vi "diagnose_status.vi"(5 "RMS mismatch":sgl, 7 "Repair count":i32, 8 "Axis positions":sgl[][](array[numeric]), 9 "Sum amplitudes":sgl[][](array[numeric]), 11 "Match error":sgl[](array[numeric])) -> (0 "Position valid":bool)   [LabVIEW 2014]
panel:
  in  "Warn RMS mismatch (volts)":sgl=0.015 format="%#_3p"
  in  "Max RMS mismatch (volts)":sgl=0.03 format="%#_3p"
  in  "Max repair count":i32=30
  in  "Max axis position":sgl=0.75
  in  "Max match error":sgl=500.0
  in  "Min amplitude":sgl=0.02
  # "Parameters:"
  # "This sets the maximum acceptable matching error between the two rays (in microns)."
  # "If impulse repair count or RMS mismatch (signal + noise) exceeds these thresholds on a single block, then the status is invalid."
  # "This sets the minimum acceptable signal amplitude."
  # "This sets the maximum acceptable axis position as a fraction of full scale."
  # "We warn if there are any impulse repairs or if the max per-block RMS mismatch exceeds this threshold."
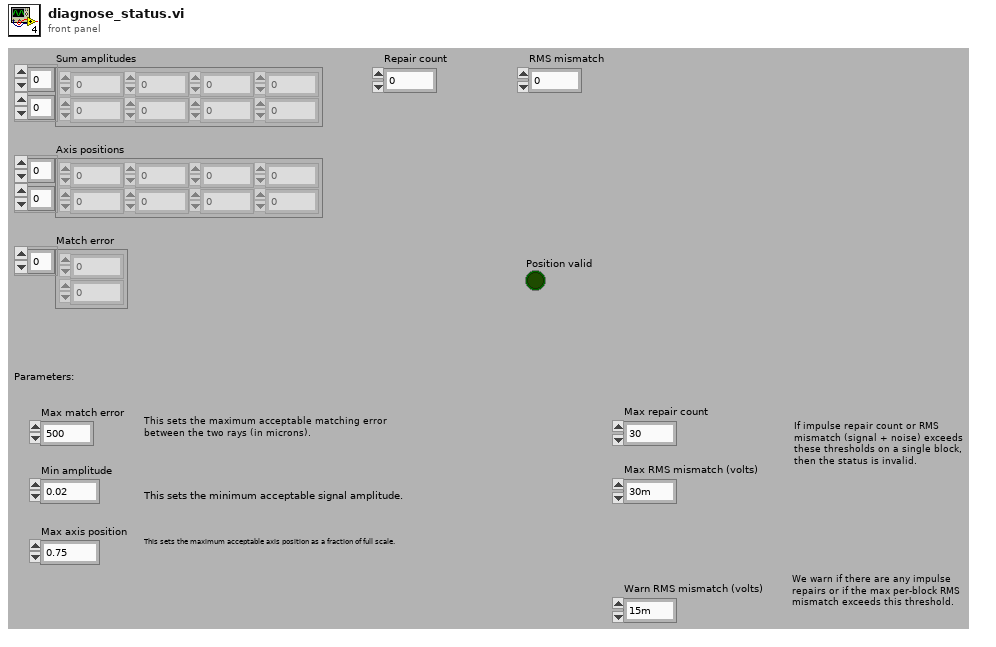
[diagram p1: front panel]
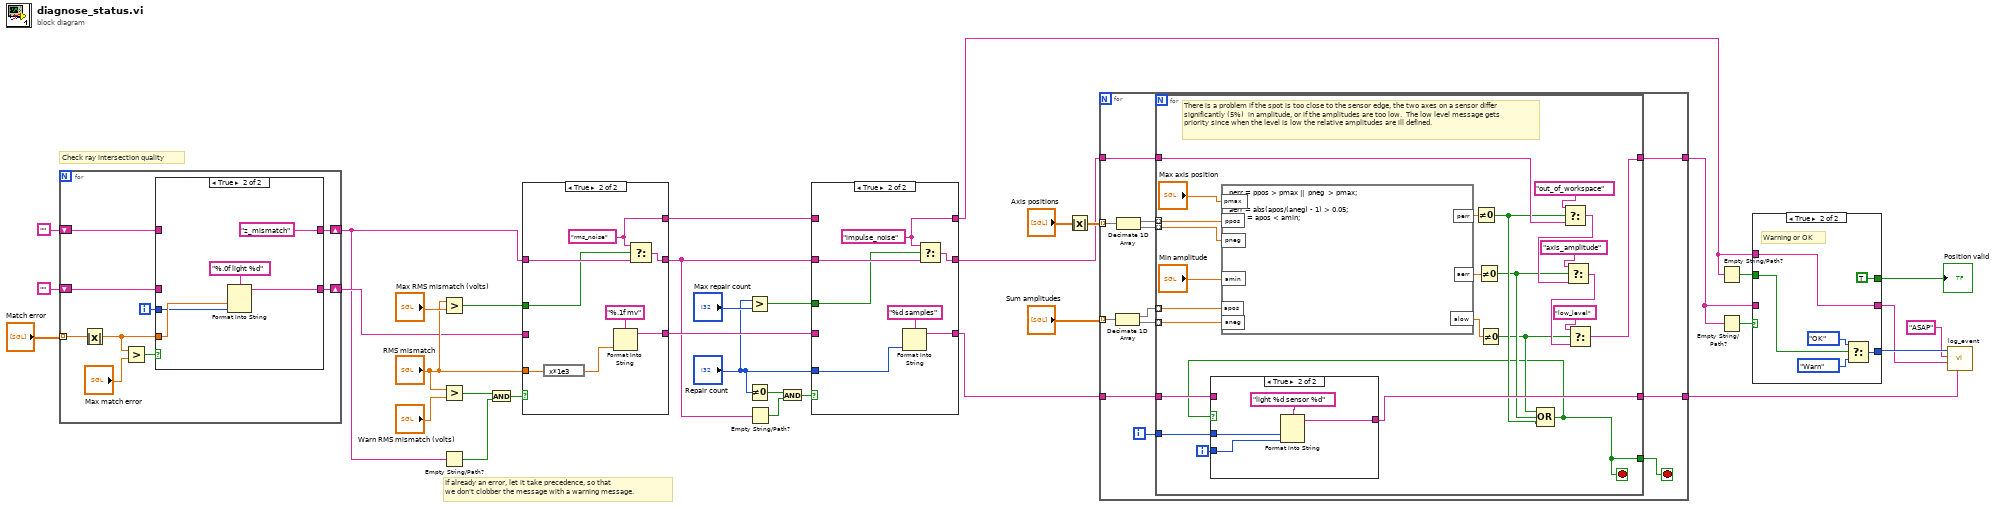
[diagram p0: block diagram]
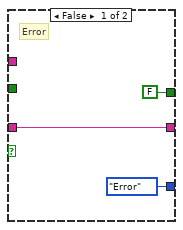
[diagram p2: hidden frame]
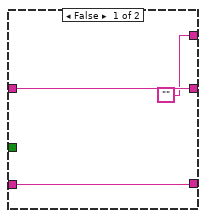
[diagram p4: hidden frame]
diagram:
  # "If already an error, let it take precedence, so that\nwe don't clobber the message with a warning message."
  # "Check ray intersection quality"
  n1 = for {
    shift-right: [w41] -> w17
    shift-left: "" -> [w42]
    tunnel: "Match error" -> [w38] mode=indexing
    shift-right: [w36] -> w9
    shift-left: "" -> [w37]
    i -> [w40]
    n2 = Absolute Value(x=w38) -> (abs(x)=w39:sgl)
    n3 = Greater?(x=w39, y="Max match error") -> (0:w43:bool)
    n4 = case shown="True" w43 {
      tunnel: w42 -> [w46 _]
      tunnel: w40 -> [_ w47]
      tunnel: w39 -> [_ w48]
      tunnel: [w46 w50] -> w41
      tunnel: w37 -> [w45 _]
      tunnel: [w45 "z_mismatch" ("format string")] -> w36
      frame False {
      }
      frame True {
        n5 = Format Into String(format string="%.0f light %d", w48, w47) -> (resulting string=w50:string)  [unwired: 2 in, 1 out]
      }
    }
  }
  n6 = Greater?(x="RMS mismatch", y="Max RMS mismatch (volts)") -> (0:w4:bool)
  n7 = Greater?(x="RMS mismatch", y="Warn RMS mismatch (volts)") -> (0:w6:bool)
  n8 = Empty String/Path?(string/path=w9) -> (empty?=w10:bool)
  n9 = And(x=w6, y=w10) -> (x .and. y?=w5:bool)
  n10 = case shown="True" w5 {
    tunnel: "RMS mismatch" -> [_ w60]
    tunnel: [w52 w61] -> w24
    tunnel: w9 -> [w54 w58]
    tunnel: ["" w56] -> w26
    tunnel: w4 -> [_ w57]
    tunnel: [w54 w55] -> w12
    tunnel: w17 -> [w52 _]
    frame False {
    }
    frame True {
      w56 = "rms_noise"
      n11 = expression code="x*1e3"(w60) -> (w59:sgl)
      n12 = Format Into String(format string="%.1f mv", w59) -> (resulting string=w61:string)  [unwired: 2 in, 1 out]
      n13 = Select(t=w56, s=w57, f=w58) -> (s? t:f=w55:string)
    }
  }
  n14 = Greater?(x="Repair count", y="Max repair count") -> (0:w7:bool)
  n15 = Not Equal To 0?(x="Repair count") -> (x != 0?=w8:bool)
  n16 = Empty String/Path?(string/path=w12) -> (empty?=w11:bool)
  n17 = And(x=w8, y=w11) -> (x .and. y?=w1:bool)
  n18 = case shown="True" w1 {
    tunnel: "Repair count" -> [_ w66]
    tunnel: [w65 w71] -> w14
    tunnel: w12 -> [w64 w70]
    tunnel: [w63 w68] -> w3
    tunnel: w24 -> [w65 _]
    tunnel: w7 -> [_ w69]
    tunnel: [w64 w67] -> w13
    tunnel: w26 -> [w63 _]
    frame False {
    }
    frame True {
      w68 = "impulse_noise"
      n19 = Format Into String(format string="%d samples", w66) -> (resulting string=w71:string)  [unwired: 2 in, 1 out]
      n20 = Select(t=w68, s=w69, f=w70) -> (s? t:f=w67:string)
    }
  }
  n21 = Absolute Value(x="Axis positions") -> (abs(x)=w32:sgl[][])
  n22 = for {
    tunnel: "Sum amplitudes" -> [w84] mode=indexing
    tunnel: w32 -> [w78] mode=indexing
    tunnel: w14 -> [w81]
    tunnel: [w79] -> w15
    tunnel: w13 -> [w75]
    tunnel: [w74] -> w16
    i -> [w80]
    stop <- w73 stop-if-true
    n23 = Decimate 1D Array(w84) -> (w83:sgl[], w82:sgl[])
    n24 = Decimate 1D Array(w78) -> (w77:sgl[], w76:sgl[])
    n25 = for {
      tunnel: w83 -> [w108] mode=indexing
      tunnel: w82 -> [w107] mode=indexing
      tunnel: w80 -> [w100]
      tunnel: w77 -> [w96] mode=indexing
      tunnel: w76 -> [w95] mode=indexing
      tunnel: [w85] -> w73
      tunnel: w81 -> [w101]
      tunnel: [w98] -> w79
      tunnel: w75 -> [w90]
      tunnel: [w89] -> w74
      i -> [w99]
      stop <- w85 stop-if-true
      # "There is a problem if the spot is too close to the sensor edge, the two axes on a sensor differ significantly (5%)  in amplitude, or if the amplitudes are too low.  The low level message gets priority since when the level is low the relative amplitudes are ill defined."
      n26 = formula code="perr = ppos > pmax ||  pneg  > pmax;\n\naerr = abs(apos/(aneg) - 1) > 0.05;\nalow = apos < amin;"("apos"=w108, "aneg"=w107, "amin"="Min amplitude", "ppos"=w96, "pneg"=w95, "pmax"="Max axis position") -> ("alow"=w102:dbl, "aerr"=w105:dbl, "perr"=w91:dbl)
      n27 = Not Equal To 0?(x=w91) -> (x != 0?=w88:bool)
      n28 = Not Equal To 0?(x=w105) -> (x != 0?=w87:bool)
      n29 = Not Equal To 0?(x=w102) -> (x != 0?=w86:bool)
      n30 = Compound Arithmetic op=OR(w86, w87, w88) -> (w85:bool)
      n31 = case shown="True" w85 {
        tunnel: w101 -> [w109 _]
        tunnel: w100 -> [_ w112]
        tunnel: w99 -> [_ w111]
        tunnel: [w109 w110] -> w98
        frame False {
        }
        frame True {
          n32 = Format Into String(format string="light %d sensor %d", w112, w111) -> (resulting string=w110:string)  [unwired: 2 in, 1 out]
        }
      }
      n33 = Select(t="out_of_workspace", s=w88, f=w90) -> (s? t:f=w92:string)
      n34 = Select(t="axis_amplitude", s=w87, f=w92) -> (s? t:f=w97:string)
      n35 = Select(t="low_level", s=w86, f=w97) -> (s? t:f=w89:string)
    }
  }
  n36 = Empty String/Path?(string/path=w3) -> (empty?=w2:bool)
  n37 = Empty String/Path?(string/path=w16) -> (empty?=w23:bool)
  n38 = case shown="True" w23 {
    tunnel: w16 -> [w116 _]
    tunnel: w3 -> [_ w120]
    tunnel: w2 -> [_ w118]
    tunnel: [w116 w120] -> w20
    tunnel: [enum16{"OK", "Debug", "Warn", "Error"}."Error" ("Severity") w119] -> w22
    tunnel: [FALSE TRUE] -> w18
    frame False {
      # "Error"
    }
    frame True {
      # "Warning or OK"
      n39 = Select(t=enum16{"OK", "Debug", "Warn", "Error"}."OK" ("Severity"), s=w118, f=enum16{"OK", "Debug", "Warn", "Error"}."Warn" ("Severity")) -> (s? t:f=w119:enum16{"OK", "Debug", "Warn", "Error"})
    }
  }
  "Position valid" <- w18
  n40 = call "log_event.vi"("Message"=w15, "State"=w20, "Facility"="ASAP", "Severity"=w22) -> ()  [unwired: 7 in, 1 out]
